vi "bar_to_pascal.vi"() -> ()   [LabVIEW 2020]
panel:
  in  "Bar":dbl(slide) scale=0.0..10.0
  out "Pascal\nKps":dbl(knob) scale=0.0..1000.0
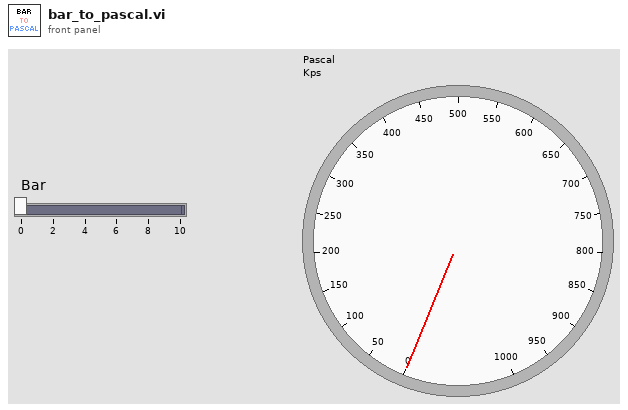
[diagram p1: front panel]
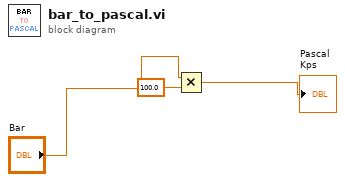
[diagram p0: block diagram]
diagram:
  n1 = Multiply(x="Bar", y=100.0) -> (x*y=→"Pascal\nKps":dbl)
